vi "SenoFPGA.vi"(8 "Fase Inicial":fxp<+,27,1>, 9 "Factor de Ajuste":fxp<+/-,32,2>=1.0, 10 "Modulacion T001":fxp<+/-,16,1>, 11 "Tasa de Incremento de Fase":fxp<+,27,0>=0.00020000338554382324) -> (2 "Sine Wave":fxp<+/-,32,2>)   [LabVIEW 2020]
uses:
  <vilib>/rvi/FXPMathLib/FxpSinAndCos/subVIs/nifxpmath_SinAndCos_SimConfig.ctl
  <vilib>/rvi/FXPMathLib/FxpSinAndCos/simVIs/DllFxpSinAndCosTemp_sub.vi
  <vilib>/rvi/FXPMathLib/FxpAdd/XNode/nifxpmath_Add.xnode
  <vilib>/rvi/FXPMathLib/FxpSinAndCos/XNode/nifxpmath_SinAndCos.xnode
  <vilib>/rvi/FXPMathLib/FxpMul/XNode/nifxpmath_Multiplier.xnode
  <vilib>/rvi/FXPMathLib/sim/FxpSim.dll
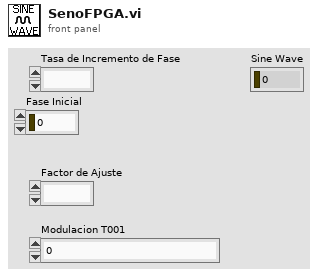
[diagram p1: front panel]
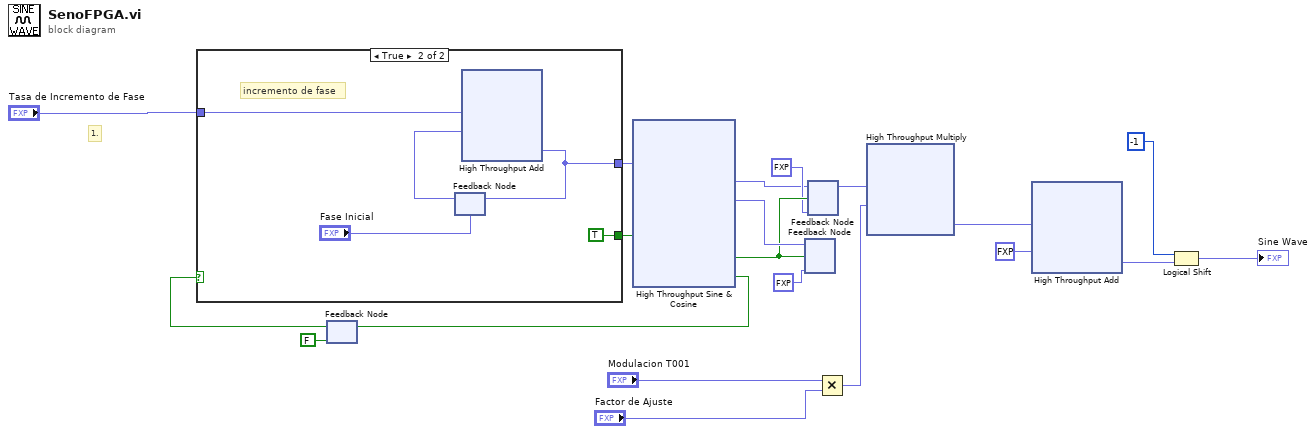
[diagram p0: block diagram]
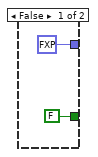
[diagram p2: hidden frame]
diagram:
  # "1."
  n1 = feedback #1(FALSE ("ready for input")) -> (w2:bool)
  n2 = case shown="True" w2 {
    tunnel: "Tasa de Incremento de Fase" -> [_ w27]
    tunnel: [fxp<+/-,16,1> 0.0 ("x+y") w24] -> w4
    tunnel: [FALSE TRUE] -> w3
    frame False {
    }
    frame True {
      # "incremento de fase"
      n3 = feedback #2("Fase Inicial") -> (w25:fxp<+,27,1>)
      n4 = xnode ("High Throughput Add")("x"=w27, "y"=w25) -> ("x+y"=w24:fxp<+,27,1>)
      n5 = feedback-in #2(w24) -> ()
    }
  }
  n6 = xnode "High Throughput Sine & Cosine"("x (pi)"=w4, "input valid"=w3) -> ("sin(x)"=w6:fxp<+/-,16,2>, "cos(x)"=w14:fxp<+/-,16,2>, "output valid"=w13:bool, "ready for input"=w5:bool)  [unwired: 1 in]
  n7 = feedback-in #1(w5) -> ()
  n8 = feedback #3(fxp<+/-,16,2> 0.0 ("cos(x)")) -> ()  [unwired: 1 in]
  n9 = feedback-in #3(w14, w13) -> ()
  n10 = feedback #4(fxp<+/-,16,2> 0.0 ("sin(x)")) -> (w7:fxp<+/-,16,2>)
  n11 = feedback-in #4(w6, w13) -> ()
  n12 = Multiply(x="Modulacion T001", y="Factor de Ajuste") -> (x*y=w16:fxp<+/-,48,3>)
  n13 = xnode ("High Throughput Multiply")("x"=w7, "y"=w16) -> ("x*y"=w11:fxp<+/-,32,2>)
  n14 = xnode ("High Throughput Add")("x"=w11, "y"=fxp<+/-,16,2> 1.0) -> ("x+y"=w9:fxp<+/-,32,2>)
  n15 = Logical Shift(y=i16 -1, x=w9) -> (x << y=→"Sine Wave":fxp<+/-,32,2>)
